vi "MoistureSensorReset.vi"(0 "GEA2 Reference In":refnum<k24>, 11 "Error In":errorcluster) -> (4 "GEA2 Reference Out":refnum<k24>, 6 "Pass/Fail?":bool, 8 "Report Text":string, 15 "Error Out":errorcluster)   [LabVIEW 2023]
uses:
  D:/Common/LabVIEW GEA2 Toolkit/source/GEA3 DLL Source/GeaCommunication.dll
  Common/LabVIEW GEA2 Toolkit/source/GEA3 DLL Source/GeaCommunication.dll
  Common/LabVIEW GEA2 Toolkit/GEA3/type defs/Source_Destination.ctl
  Common/LabVIEW GEA2 Toolkit/GEA3/type defs/ERD Write Data In.ctl
  Common/LabVIEW GEA2 Toolkit/GEA3/type defs/Data Type.ctl
  Common/LabVIEW GEA2 Toolkit/GEA3/type defs/ERD Read Data In.ctl
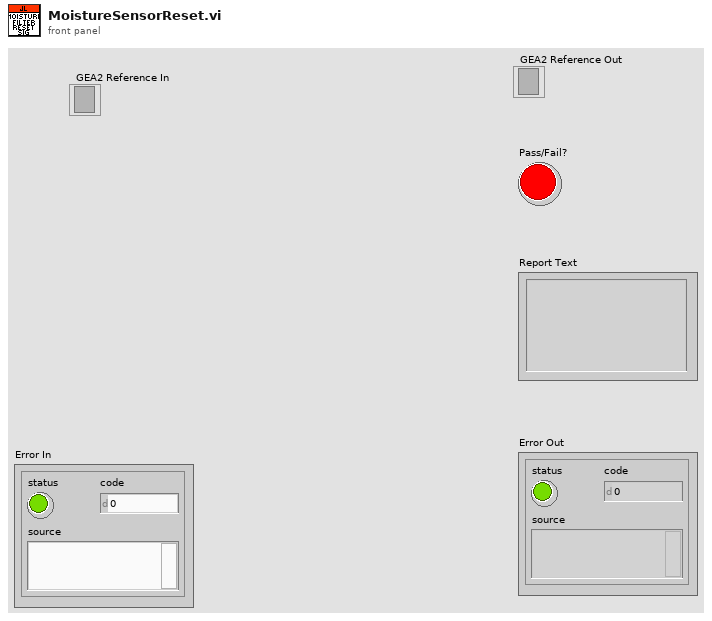
[diagram p1: front panel]
types:
  T1 = typedef "ERD Read Data In.ctl" = cluster{"ERD Number":u16, "Data Type":enum16{"string", "boolean", "uint8_t", "uint16_t", "uint32_t", "uint64_t", "int8_t", "int16_t", "int32_t", "int64_t"}}
  T2 = typedef "ERD Write Data In.ctl" = cluster{"ERD Number":u16, "Data Type":T3, "Data":string}
  T3 = typedef "Data Type.ctl" = enum16{"string", "boolean", "uint8_t", "uint16_t", "uint32_t", "uint64_t", "int8_t", "int16_t", "int32_t", "int64_t"}
  T4 = typedef "Source_Destination.ctl" = cluster{"Source":u8, "Destination":u8}
  T5 = typedef "ERD Read Data Out.ctl" = cluster{"ERD Number":u16, "Data":string}
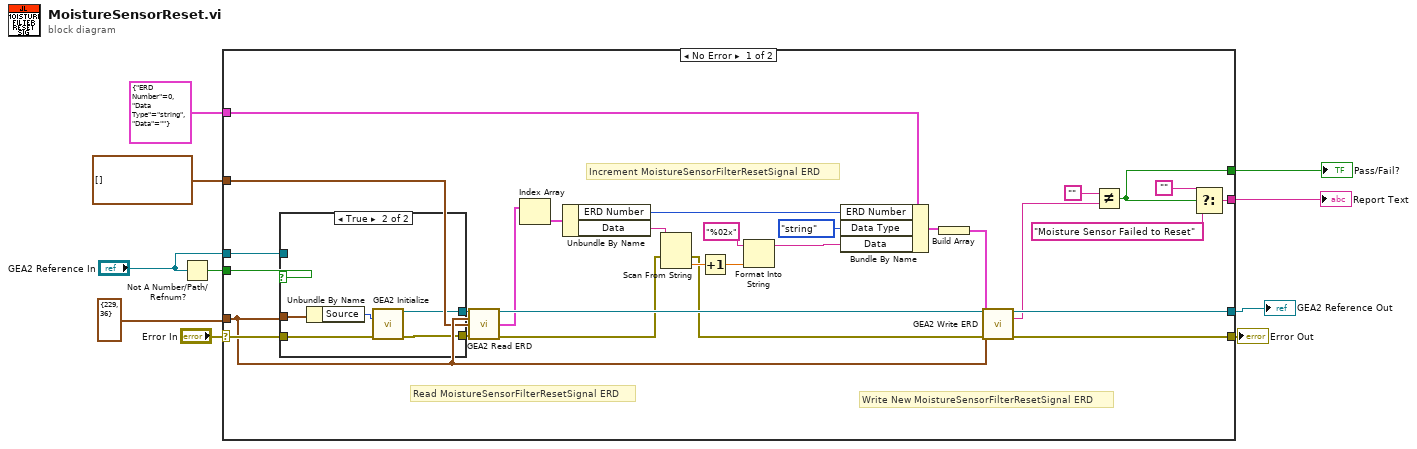
[diagram p0: block diagram]
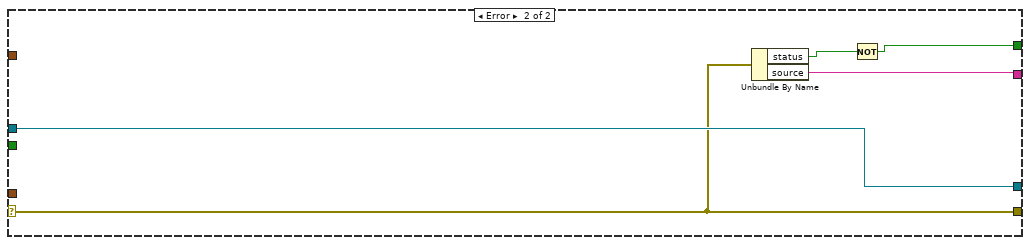
[diagram p3: hidden frame]
diagram:
  n1 = Not A Number/Path/Refnum?(number/path/refnum="GEA2 Reference In") -> (NaN/Path/Refnum?=w10:bool)
  n2 = case shown="No Error" "Error In" {
    selector: "Error In" -> [w24 w51]
    tunnel: [w39 w52] -> w2
    tunnel: w10 -> [w26 _]
    tunnel: "GEA2 Reference In" -> [w25 w52]
    tunnel: T4 {"Source"=229, "Destination"=36} ("GEA Inputs") -> [w21 _]
    tunnel: T2 {"ERD Number"=0, "Data Type"=enum."string", "Data"=""} ("ERD Write Data In") -> [w22 _]
    tunnel: T1[] [] ("Read ERD List") -> [w20 _]
    tunnel: [w17 w51] -> w5
    tunnel: [w16 w48] -> w3
    tunnel: [w14 w50] -> w4
    frame No Error {
      # "Write New MoistureSensorFilterResetSignal ERD"
      # "Increment MoistureSensorFilterResetSignal ERD"
      # "Read MoistureSensorFilterResetSignal ERD"
      n3 = case shown="True" w26 {
        tunnel: w21 -> [_ w47]
        tunnel: [w42 w45] -> w28
        tunnel: w25 -> [w42 _]
        tunnel: w24 -> [w41 w44]
        tunnel: [w41 w43] -> w23
        frame False {
        }
        frame True {
          n4 = Unbundle By Name(w47) -> ("Source"=w46:u8)
          n5 = call "GEA2 Initialize.vi"("Source Address"=w46, "error in"=w44) -> ("GEA2 Reference Out"=w45:refnum<k24>, "error out"=w43:errorcluster)  [unwired: 11 in, 1 out]
        }
      }
      n6 = call "GEA2 Read ERD.vi"("GEA2 Reference In"=w28, "GEA Inputs"=w21, "Read ERD List"=w20, "Error In"=w23) -> ("GEA2 Reference Out"=w40:refnum<k24>, "ERD Data Out"=w38:T5[], "Error Out"=w12:errorcluster)  [unwired: 8 in, 1 out]
      n7 = Index Array(array=w38) -> (element=w37:T5)  [unwired: 1 in]
      n8 = Unbundle By Name(w37) -> ("ERD Number"=w36:u16, "Data"=w34:string)
      n9 = Scan From String(input string=w34, error in=w12) -> (error out=w11:errorcluster, output 1=w33:dbl)  [unwired: 3 in, 2 out]
      n10 = Increment(x=w33) -> (x+1=w32:dbl)
      n11 = Format Into String(format string="%02x", w32) -> (resulting string=w31:string)  [unwired: 2 in, 1 out]
      n12 = Bundle By Name(cluster=w22, "ERD Number"=w36, "Data Type"=Data_Type."string", "Data"=w31) -> (w30:T2)
      n13 = Build Array(w30) -> (w29:T2[])
      n14 = call "GEA2 Write ERD.vi"("GEA2 Reference In"=w40, "GEA Inputs"=w21, "Write ERD List"=w29, "Error In"=w11) -> ("GEA2 Reference Out"=w39:refnum<k24>, "Raw Data Out"=w15:string, "Error Out"=w17:errorcluster)  [unwired: 9 in]
      n15 = Not Equal?(x="", y=w15) -> (x != y?=w16:bool)
      n16 = Select(t="", s=w16, f="Moisture Sensor Failed to Reset") -> (s? t:f=w14:string)
    }
    frame Error {
      n17 = Unbundle By Name(w51) -> ("status"=w49:bool, "source"=w50:string)
      n18 = Not(x=w49) -> (.not. x?=w48:bool)
    }
  }
  "GEA2 Reference Out" <- w2
  "Error Out" <- w5
  "Report Text" <- w4
  "Pass/Fail?" <- w3
